vi "Rinocloud_JSON_encoder.vi"(0 "Metadata":T2, 1 "Extra metadata array":T1(array[cluster])=[{"Attribute"="", "Value"="", "Data type"=enum."<null>"}, {"Attribute"="Amplitude", "Value"="10", "Data type"=enum."<null>"}], 2 "parent ID":string, 3 "error in (no error)":errorcluster, 4 "self ID":string) -> (5 "JSON payload":string, 6 "error out":errorcluster)   [LabVIEW 2013]
uses:
  i3 JSON/JSON Generation/Create Value Files/Create Value - Object.vi
  i3 JSON/JSON Generation/Add Object Parameter Files/Add Object Parameter - String.vi
  i3 JSON/JSON Generation/Add Object Parameter Files/Add Object Parameter - 1D Array String.vi
  i3 JSON/JSON Generation/Add Object Parameter Files/Add Object Parameter - Numeric.vi
  i3 JSON/JSON Generation/Add Object Parameter Files/Add Object Parameter - 1D Array Double.vi
  i3 JSON/JSON Generation/Add Object Parameter Files/Add Object Parameter - Data JSON string.vi
  i3 JSON/i3-json.lvlib
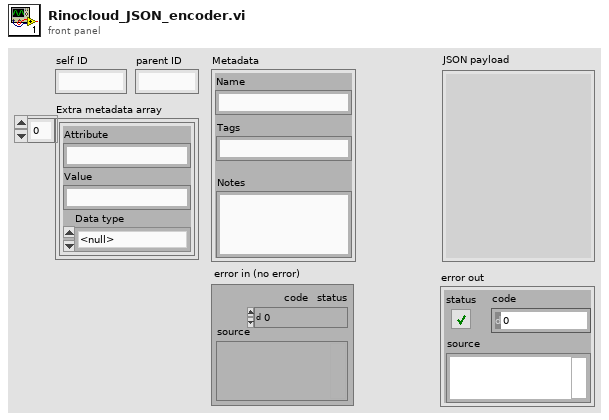
[diagram p1: front panel]
types:
  T1 = cluster{"Attribute":string, "Value":string, "Data type":enum16{"Numeric", "String", "1D array of strings", "1D array of doubles", "Data JSON string", "<null>"}}[]
  T2 = cluster{"Name":string, "Notes":string, "Tags":string}
  T3 = enum16{"Numeric", "String", "1D array of strings", "1D array of doubles", "Data JSON string", "<null>"}
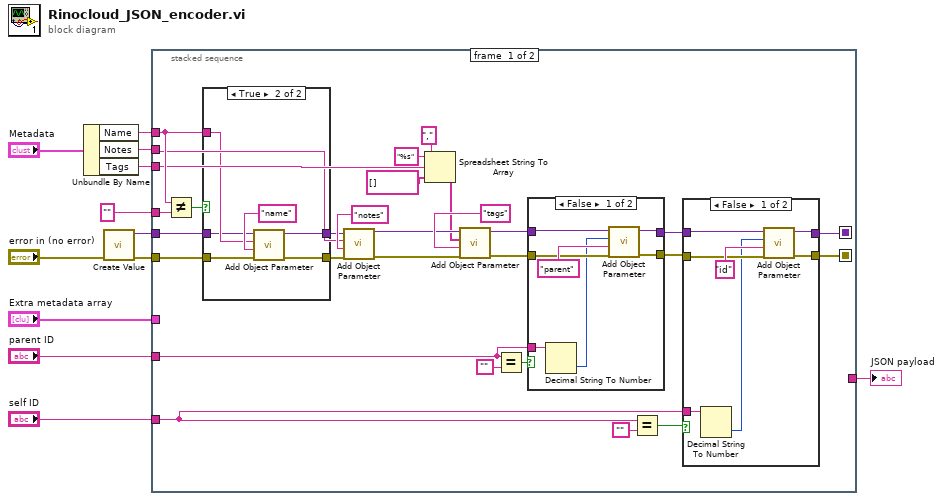
[diagram p0: block diagram]
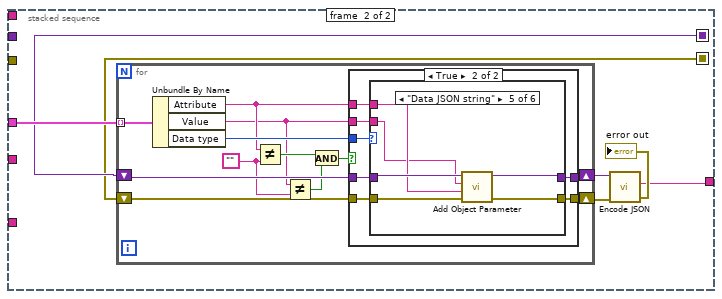
[diagram p5: hidden frame]
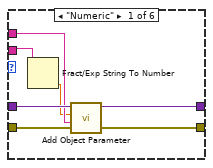
[diagram p7: hidden frame]
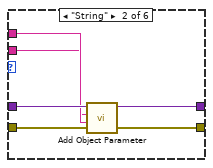
[diagram p8: hidden frame]
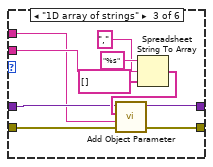
[diagram p9: hidden frame]
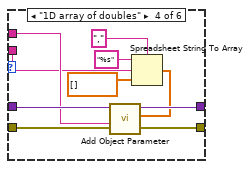
[diagram p10: hidden frame]
diagram:
  n1 = Unbundle By Name("Metadata") -> ("Name"=w8:string, "Notes"=w6:string, "Tags"=w7:string)
  n2 = call-poly "Create Value.vi"("error in (no error)"="error in (no error)") -> ("error out"=w4:errorcluster, "JSON Tree"=w11:variant)  [unwired: 9 in]
  n3 = stacked-sequence {
    seq-local: [w17 _] -> [_ w70]
    seq-local: [w16 _] -> [_ w69]
    tunnel: w8 -> [w39 _]
    tunnel: w6 -> [w28 _]
    tunnel: w7 -> [w31 _]
    tunnel: w11 -> [w40 _]
    tunnel: "" ("y") -> [w38 _]
    tunnel: "Extra metadata array" -> [_ w74]
    tunnel: [_ w68] -> w10
    tunnel: w4 -> [w37 _]
    tunnel: "parent ID" -> [w20 _]
    tunnel: "self ID" -> [w13 _]
    frame #0 {
      n4 = Not Equal?(x=w39, y=w38) -> (x != y?=w41:bool)
      n5 = case shown="True" w41 {
        tunnel: w40 -> [w61 w65]
        tunnel: w39 -> [_ w66]
        tunnel: [w61 w64] -> w30
        tunnel: w37 -> [w60 w63]
        tunnel: [w60 w62] -> w29
        frame False {
        }
        frame True {
          n6 = call-poly "Add Object Parameter.vi"("error in (no error)"=w63, "Name"="name", "String"=w66, "JSON Tree in (JSON Object)"=w65) -> ("error out"=w62:errorcluster, "JSON Tree out (JSON Object)"=w64:variant)  [unwired: 6 in]
        }
      }
      n7 = call-poly "Add Object Parameter.vi"("error in (no error)"=w29, "Name"="notes", "String"=w28, "JSON Tree in (JSON Object)"=w30) -> ("error out"=w26:errorcluster, "JSON Tree out (JSON Object)"=w27:variant)  [unwired: 6 in]
      n8 = Spreadsheet String To Array(delimiter (Tab)=",", format string="%s", spreadsheet string=w31, array type (2D Dbl)=string[] [] ("Array")) -> (array=w25:string[])
      n9 = call-poly "Add Object Parameter.vi"("error in (no error)"=w26, "Name"="tags", "1D String"=w25, "JSON Tree in (JSON Object)"=w27) -> ("error out"=w22:errorcluster, "JSON Tree out (JSON Object)"=w23:variant)  [unwired: 6 in]
      n10 = Equal?(x=w20, y="") -> (x = y?=w21:bool)
      n11 = case shown="False" w21 {
        tunnel: w23 -> [w55 w59]
        tunnel: [w56 w59] -> w19
        tunnel: [w57 w58] -> w18
        tunnel: w22 -> [w53 w58]
        tunnel: w20 -> [w52 _]
        frame False {
          n12 = Decimal String To Number(string=w52) -> (number=w51:i32)  [unwired: 2 in, 1 out]
          n13 = call-poly "Add Object Parameter.vi"("error in (no error)"=w53, "Name"="parent", "Numeric"=w51, "JSON Tree in (JSON Object)"=w55) -> ("error out"=w57:errorcluster, "JSON Tree out (JSON Object)"=w56:variant)  [unwired: 6 in]
        }
        frame True {
        }
      }
      n14 = Equal?(x=w13, y="") -> (x = y?=w14:bool)
      n15 = case shown="False" w14 {
        tunnel: w19 -> [w46 w50]
        tunnel: [w47 w50] -> w17
        tunnel: [w48 w49] -> w16
        tunnel: w18 -> [w44 w49]
        tunnel: w13 -> [w43 _]
        frame False {
          n16 = Decimal String To Number(string=w43) -> (number=w42:i32)  [unwired: 2 in, 1 out]
          n17 = call-poly "Add Object Parameter.vi"("error in (no error)"=w44, "Name"="id", "Numeric"=w42, "JSON Tree in (JSON Object)"=w46) -> ("error out"=w48:errorcluster, "JSON Tree out (JSON Object)"=w47:variant)  [unwired: 6 in]
        }
        frame True {
        }
      }
    }
    frame #1 {
      n18 = for {
        tunnel: w74 -> [w86] mode=indexing
        shift-right: [w81] -> w73
        shift-left: w70 -> [w82]
        shift-right: [w83] -> w71
        shift-left: w69 -> [w84]
        w76 = ""
        n19 = Unbundle By Name(w86) -> ("Attribute"=w80:string, "Value"=w75:string, "Data type"=w85:T3)
        n20 = Not Equal?(x=w80, y=w76) -> (x != y?=w78:bool)
        n21 = Not Equal?(x=w75, y=w76) -> (x != y?=w77:bool)
        n22 = And(x=w78, y=w77) -> (x .and. y?=w79:bool)
        n23 = case shown="True" w79 {
          tunnel: w85 -> [_ w95]
          tunnel: w84 -> [w87 w94]
          tunnel: [w87 w93] -> w83
          tunnel: w82 -> [w88 w92]
          tunnel: [w88 w91] -> w81
          tunnel: w80 -> [_ w90]
          tunnel: w75 -> [_ w89]
          frame False {
          }
          frame True {
            n24 = case shown="\"Data JSON string\"" w95 {
              tunnel: w94 -> [w102 w105 w113 w126 w134 w135]
              tunnel: [w101 w106 w109 w124 w133 w135] -> w93
              tunnel: w92 -> [w100 w108 w114 w127 w132 w136]
              tunnel: [w99 w107 w110 w125 w131 w136] -> w91
              tunnel: w90 -> [w98 w104 w111 w123 w130 _]
              tunnel: w89 -> [w96 w103 w112 w122 w129 _]
              frame "Numeric" {
                n25 = Fract/Exp String To Number(string=w96) -> (number=w97:dbl)  [unwired: 3 in, 1 out]
                n26 = call-poly "Add Object Parameter.vi"("error in (no error)"=w102, "Name"=w98, "Numeric"=w97, "JSON Tree in (JSON Object)"=w100) -> ("error out"=w101:errorcluster, "JSON Tree out (JSON Object)"=w99:variant)  [unwired: 6 in]
              }
              frame "String" {
                n27 = call-poly "Add Object Parameter.vi"("error in (no error)"=w105, "Name"=w104, "String"=w103, "JSON Tree in (JSON Object)"=w108) -> ("error out"=w106:errorcluster, "JSON Tree out (JSON Object)"=w107:variant)  [unwired: 6 in]
              }
              frame "1D array of strings" {
                n28 = Spreadsheet String To Array(delimiter (Tab)=",", format string="%s", spreadsheet string=w112, array type (2D Dbl)=string[] [] ("Array")) -> (array=w116:string[])
                n29 = call-poly "Add Object Parameter.vi"("error in (no error)"=w113, "Name"=w111, "1D String"=w116, "JSON Tree in (JSON Object)"=w114) -> ("error out"=w109:errorcluster, "JSON Tree out (JSON Object)"=w110:variant)  [unwired: 6 in]
              }
              frame "1D array of doubles" {
                n30 = Spreadsheet String To Array(delimiter (Tab)=",", format string="%s", spreadsheet string=w122, array type (2D Dbl)=dbl[] []) -> (array=w119:dbl[])
                n31 = call-poly "Add Object Parameter.vi"("error in (no error)"=w126, "Name"=w123, "1D Double"=w119, "JSON Tree in (JSON Object)"=w127) -> ("error out"=w124:errorcluster, "JSON Tree out (JSON Object)"=w125:variant)  [unwired: 6 in]
              }
              frame "Data JSON string" {
                n32 = call-poly "Add Object Parameter.vi"("error in (no error)"=w134, "Name"=w130, "String"=w129, "JSON Tree in (JSON Object)"=w132) -> ("error out"=w133:errorcluster, "JSON Tree out (JSON Object)"=w131:variant)  [unwired: 6 in]
              }
              frame "<null>", Default {
              }
            }
          }
        }
      }
      n33 = call "Encode JSON.vi"("error in (no error)"=w71, "JSON Tree"=w73) -> ("error out"=→"error out":errorcluster, "String"=w68:string)  [unwired: 4 in]
    }
  }
  "JSON payload" <- w10
